vi "AutoFollowAbsoluteTrajectory.vi"(8 "error in (no error)":errorcluster, 9 "TimeOut (s)":dbl, 11 "Trajectory":T1 {"States"."POSE"."ROTATION"."SIN" format="%13.4f"; "States"."POSE"."ROTATION"."COS" format="%13.4f"; "States"."POSE"."ROTATION"."VALUE" format="%13.4f"; "States"."POSE"."TRANSLATION"."Y" format="%14.3f"; "States"."POSE"."TRANSLATION"."X" format="%14.3f"; "TotalTImeSecs" format="%20.3f"}) -> (0 "error out":errorcluster)   [LabVIEW 2023]
doc: "Wrapper class for drive straight"
uses:
  <vilib>/Rock Robotics/WPI/ThirdParty/JAS_Junk/TrajLib/TypeDef/TRAJECTORY.ctl
  <vilib>/Rock Robotics/WPI/ThirdParty/JAS_Junk/TrajLib/TypeDef/TRAJ_STATE.ctl
  <vilib>/Rock Robotics/WPI/ThirdParty/JAS_Junk/TrajLib/TypeDef/POSE2D.ctl
  <vilib>/Rock Robotics/WPI/ThirdParty/JAS_Junk/TrajLib/TypeDef/TRANSLATION2D.ctl
  <vilib>/Rock Robotics/WPI/ThirdParty/JAS_Junk/TrajLib/TypeDef/ROTATION2D.ctl
  <vilib>/Utility/semaphor.llb/Obtain Semaphore Reference.vi
  <vilib>/Rock Robotics/WPI/ThirdParty/JAS_Junk/TrajLib/Timer_Reset.vi
  <vilib>/Rock Robotics/WPI/ThirdParty/JAS_Junk/TrajLib/Trajectory_Library.lvlib
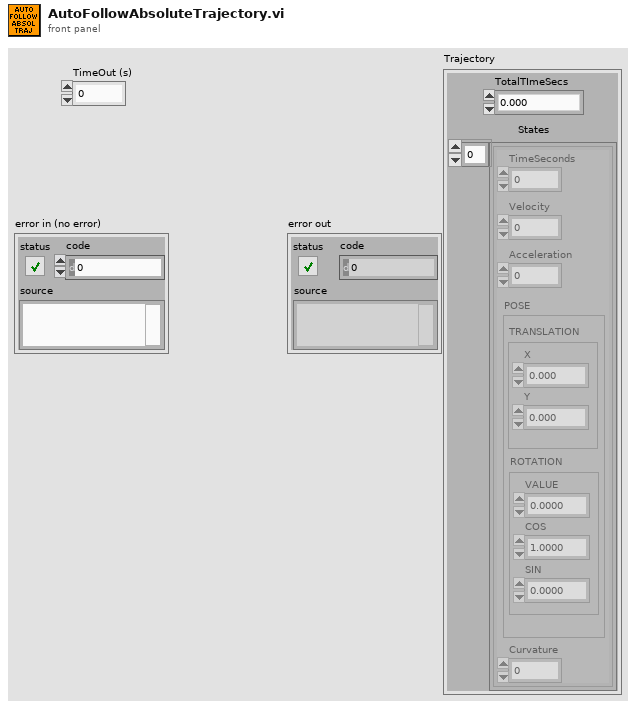
[diagram p1: front panel]
types:
  T1 = typedef "Trajectory_Library.lvlib/TRAJECTORY.ctl" = cluster{"TotalTImeSecs":dbl, "States":T2[]}
  T2 = typedef "Trajectory_Library.lvlib/TRAJ_STATE.ctl" = cluster{"TimeSeconds":dbl, "Velocity":dbl, "Acceleration":dbl, "POSE":T3, "Curvature":dbl}
  T3 = typedef "Trajectory_Library.lvlib/POSE2D.ctl" = cluster{"TRANSLATION":T4, "ROTATION":T5}
  T4 = typedef "Trajectory_Library.lvlib/TRANSLATION2D.ctl" = cluster{"X":dbl, "Y":dbl}
  T5 = typedef "Trajectory_Library.lvlib/ROTATION2D.ctl" = cluster{"VALUE":dbl, "COS":dbl, "SIN":dbl}
  T6 = typedef "Trajectory_Library.lvlib/TIMER.ctl" = cluster{"StartTime":dbl, "Accumulated TIme":dbl, "Running":bool, "semaphore":T7}
  T7 = typedef "Semaphore RefNum" = refnum<k1>
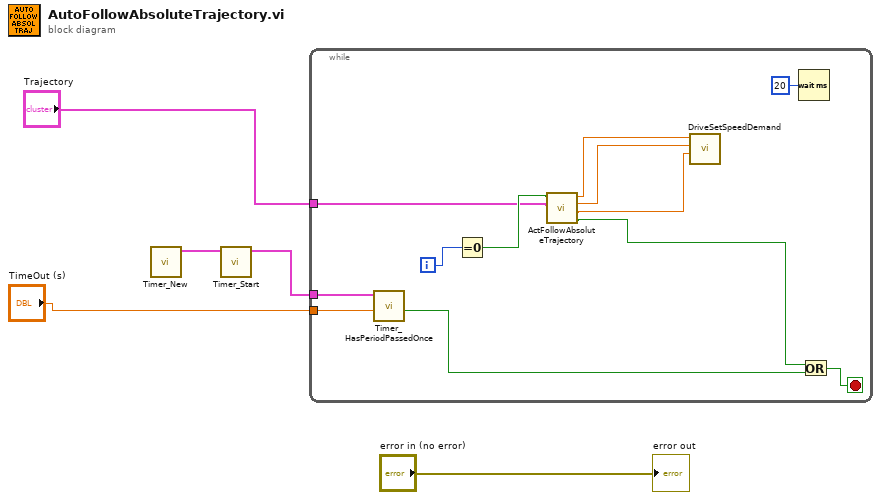
[diagram p0: block diagram]
diagram:
  n1 = call <vilib>:"Timer_New.vi"() -> ("TIMER"=w4:T6)  [unwired: 11 in]
  n2 = call <vilib>:"Timer_Start.vi"("in Timer"=w4) -> ("out Timer"=w3:T6)  [unwired: 10 in]
  n3 = while {
    tunnel: w3 -> [w16]
    tunnel: "TimeOut (s)" -> [w15]
    tunnel: "Trajectory" -> [w10]
    i -> [w17]
    stop <- w13 stop-if-true
    n4 = call <vilib>:"Timer_HasPeriodPassedOnce.vi"("Period"=w15, "in Timer"=w16) -> ("Expired"=w14:bool)  [unwired: 7 in, 2 out]
    n5 = Equal To 0?(x=w17) -> (x = 0?=w11:bool)
    n6 = call "ActFollowAbsoluteTrajectory.vi"("Trajectory"=w10, "FirstTime"=w11) -> ("Done"=w6:bool, "ASpeedDemand"=w7:dbl, "YSpeedDemand"=w8:dbl, "XSpeedDemand"=w9:dbl)  [unwired: 6 in]
    n7 = call "DriveSetSpeedDemand.vi"("ASpeedDemand (d/s)"=w7, "YSpeedDemand (ft/s)"=w8, "XSpeedDemand (ft/s)"=w9) -> ()  [unwired: 9 in]
    n8 = Wait (ms)(milliseconds to wait=u32 20) -> ()  [unwired: 1 out]
    n9 = Or(x=w6, y=w14) -> (x .or. y?=w13:bool)
  }
  "error out" <- "error in (no error)"
